vi "TranslatePathSup_Array.vi"(10 "Offset":cluster{dbl, dbl}, 11 "PathSupsIn":T1[](array[typedef])) -> (3 "PathSupsOut":T1[](array[typedef]))   [LabVIEW 2014]
uses:
  TypeDefs/PathSupreme.ctl
  PSup2SCAN/Sub/VelocityProfile.ctl
  PSup2SCAN/Sub/PathCut.ctl
  PSup2SCAN/Sub/Segment.ctl
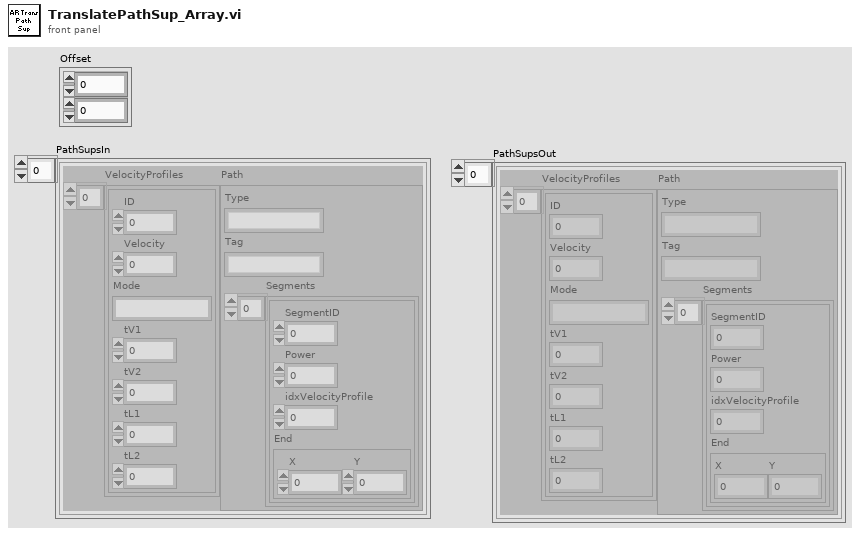
[diagram p1: front panel]
types:
  T1 = typedef "PathSupreme.ctl" = cluster{"VelocityProfiles":T2[], "Path":T3}
  T2 = typedef "VelocityProfile.ctl" = cluster{"ID":u32, "Velocity":dbl, "Mode":string, "tV1":u32, "tV2":u32, "tL1":u32, "tL2":u32}
  T3 = typedef "PathCut.ctl" = cluster{"Type":string, "Tag":string, "Segments":T4[]}
  T4 = typedef "Segment.ctl" = cluster{"SegmentID":u16, "Power":sgl, "idxVelocityProfile":u16, "End":cluster{"X":sgl, "Y":sgl}}
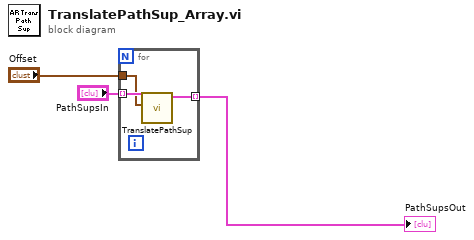
[diagram p0: block diagram]
diagram:
  n1 = for {
    tunnel: "PathSupsIn" -> [w6] mode=indexing
    tunnel: [w5] -> w2 mode=indexing
    tunnel: "Offset" -> [w4]
    n2 = call "TranslatePathSup.vi"("Offset"=w4, "PathSupreme"=w6) -> ("PathSupOut"=w5:T1)  [unwired: 9 in]
  }
  "PathSupsOut" <- w2
